vi "helper - polar plot.vi"(0 "picture":picture, 1 "desired font(Application)":T2(ring)=enum."Application Font", 2 "[user-specified font]":T3, 5 "data array [mag, phase (deg)]":cluster{"magnitude":dbl, "phase":dbl}[](array[cluster]) {"phase" format="%0.2f"; "magnitude" format="%0.2f"}, 7 "top left point(0, 0)":cluster{"x":i16, "y":i16}, 9 "dimensions (w,h)":cluster{"width":i16, "height":i16}, 11 "polar attributes":T1={"maximum"=0.0, "minimum"=0.0, "clip to min"=FALSE, "log?(F)"=FALSE, "grid color"=6710886, "plot color"=65280, "fmt and prec"={"format"=enum."Decimal", "precision"=0}, "visible section"=8} {"minimum" format="%0.2f"; "maximum" format="%0.2f"}, 12 "Lines/Points":enum16{"Lines", "Points"}(ring), 13 "Size":u16=1) -> (4 "new picture":picture)   [LabVIEW 2011]
doc: "Takes a picture and polar data and appends a picture that represents a polar graph of the data."
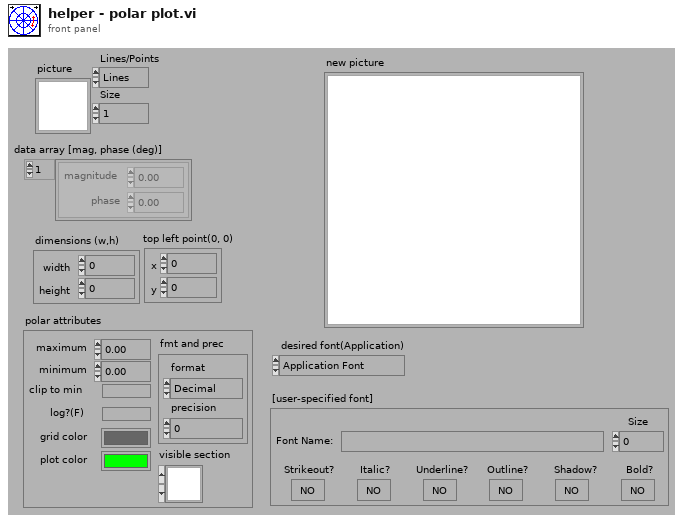
[diagram p1: front panel]
types:
  T1 = cluster{"maximum":dbl, "minimum":dbl, "clip to min":bool, "log?(F)":bool, "grid color":u32, "plot color":u32, "fmt and prec":cluster{"format":enum8{"Decimal", "Scientific", "Engineering", "Binary", "Octal", "Hex"}, "precision":u8}, "visible section":u16}
  T2 = enum16{"User-specified Font", "Application Font", "System Font", "Dialog Font"}
  T3 = cluster{"Font Name:":string, "Size":i16, "Strikeout?":bool, "Italic?":bool, "Underline?":bool, "Outline?":bool, "Shadow?":bool, "Bold?":bool}
  T4 = cluster{"left":i16, "top":i16, "right":i16, "bottom":i16}
  T5 = cluster{"pixel center":cluster{"x":i16, "y":i16}, "scale factors":cluster{"a":dbl, "b":dbl, "log?":bool}, "grid color":u32, "start angle":dbl, "end angle":dbl, "tick length":i16, "pixel radius":i32}
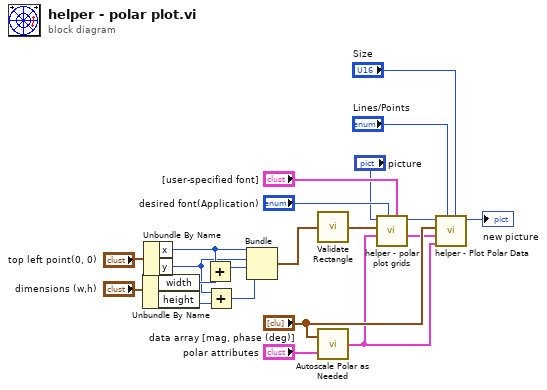
[diagram p0: block diagram]
diagram:
  n1 = Unbundle By Name("dimensions (w,h)") -> ("width"=w9:i16, "height"=w8:i16)
  n2 = Unbundle By Name("top left point(0, 0)") -> ("x"=w7:i16, "y"=w6:i16)
  n3 = Add(x=w7, y=w9) -> (x+y=w5:i16)
  n4 = Add(x=w6, y=w8) -> (x+y=w4:i16)
  n5 = Bundle("x"=w7, "y"=w6, w5, w4) -> (w3:cluster{"x":i16, "y":i16, i16, i16})  [unwired: 1 in]
  n6 = call <vilib>:"Validate Rectangle.vi"("rect"=w3) -> ("valid rect"=w12:T4)
  n7 = call <vilib>:"Autoscale Polar as Needed.vi"("polar attributes"="polar attributes", "data"="data array [mag, phase (deg)]") -> ("polar attributes"=w14:T1)
  n8 = call "helper - polar plot grids.vi"("[user-specified font]"="[user-specified font]", "desired font(Application)"="desired font(Application)", "polar attributes"=w14, "rect"=w12, "picture"="picture") -> ("grid measurements"=w13:T5, "new picture"=w15:picture)  [unwired: 5 in]
  n9 = call "helper - Plot Polar Data.vi"("Size"="Size", "Lines/Points"="Lines/Points", "polar attributes"=w14, "grid measurements"=w13, "polar data"="data array [mag, phase (deg)]", "picture"=w15) -> ("new picture"=→"new picture":picture)  [unwired: 3 in]
